vi "Pulsante.vi"() -> ()   [LabVIEW 2018]
panel:
  in  "Fondo Scala":dbl(ring)=10.0 items=["10"=10.0, "5"=5.0, "0.5  or 1"=0.5, "0.05 or 0.2"=0.05]
  in  "Fondo Scala 6x21":dbl(ring)=10.0 items=["10"=10.0, "5"=5.0, "1"=1.0, "0.2"=0.2]
  in  "Fondo Scala 6024":dbl(ring)=10.0 items=["10"=10.0, "5"=5.0, "0.5"=0.5, "0.05"=0.05]
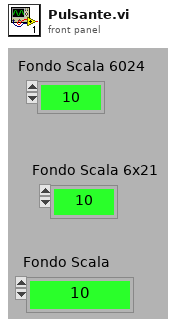
[diagram p1: front panel]
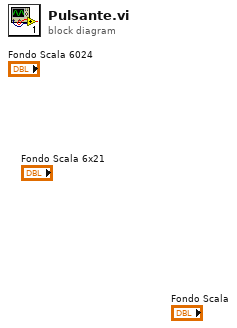
[diagram p0: block diagram]
diagram:
